vi "upload_session_start.vi"(8 "error in (no error)":errorcluster) -> (0 "error out":errorcluster, 3 "session_id":string)   [LabVIEW 2015, in "lv-dropbox.lvlib" / "v2.lvlib"]
uses:
  v2.lvlib
  private/_controls/content_type.ctl
  <vilib>/httpClient/POSTBuffer.vi
  <vilib>/httpClient/LabVIEWHTTPClient.lvlib
  lv-dropbox.lvlib
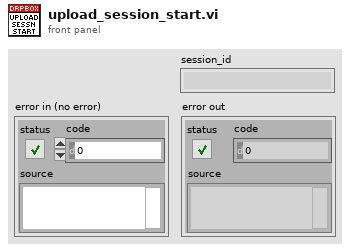
[diagram p1: front panel]
types:
  T1 = typedef "lv-dropbox.lvlib/content_type.ctl" = enum16{"<content_type>", "application/json", "application/octet-stream", "application/x-www-form-urlencoded"}
  T2 = typedef "LabVIEWHTTPClient.lvlib/ClientHandle.ctl" = refnum<k1>
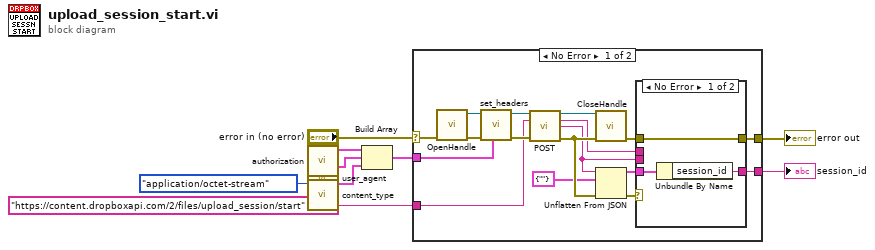
[diagram p0: block diagram]
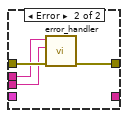
[diagram p2: hidden frame]
diagram:
  n1 = call "authorization.vi"() -> ("header"=w4:cluster{"header":string, "value":string})  [unwired: 11 in]
  n2 = call "user_agent.vi"() -> ("header"=w8:cluster{"header":string, "value":string})  [unwired: 11 in]
  n3 = call "content_type.vi"("content_type"=content_type."application/octet-stream") -> ("header"=w9:cluster{"header":string, "value":string})  [unwired: 10 in]
  n4 = Build Array(w4, w8, w9) -> (w3:cluster{"header":string, "value":string}[])
  n5 = case shown="No Error" "error in (no error)" {
    selector: "error in (no error)" -> [w20 w34]
    tunnel: w3 -> [w18 _]
    tunnel: "https://content.dropboxapi.com/2/files/upload_session/start" ("url") -> [w15 _]
    tunnel: [w10 w34] -> w1
    tunnel: [w16 _] -> w2
    frame No Error {
      n6 = call <vilib>:"OpenHandle.vi"("error in (no error)"=w20) -> ("client handle out"=w23:T2, "error out"=w17:errorcluster)  [unwired: 13 in]
      n7 = call "set_headers.vi"("header_value []"=w18, "error in (no error)"=w17, "client_handle in"=w23) -> ("error out"=w21:errorcluster, "client_handle out"=w22:T2)  [unwired: 7 in]
      n8 = call-poly <vilib>:"POST.vi"("client handle"=w22, "url"=w15, "error in (no error)"=w21) -> ("client handle out"=w24:T2, "headers"=w13:string, "body"=w12:string, "error out"=w26:errorcluster)  [unwired: 9 in]
      n9 = call <vilib>:"CloseHandle.vi"("client handle"=w24, "error in (no error)"=w26) -> ("error out"=w11:errorcluster)  [unwired: 13 in]
      n10 = Unflatten From JSON(JSON string=w12, type and defaults=cluster{"session_id":string} {"session_id"=""} ("value"), error in (no error)=w26) -> (value=w25:cluster{"session_id":string}, error out=w14:errorcluster)  [unwired: 4 in]
      n11 = case shown="No Error" w14 {
        tunnel: w25 -> [w29 _]
        tunnel: [w28 _] -> w16
        tunnel: w13 -> [_ w32]
        tunnel: w12 -> [_ w31]
        tunnel: w11 -> [w27 w33]
        tunnel: [w27 w30] -> w10
        frame No Error {
          n12 = Unbundle By Name(w29) -> ("session_id"=w28:string)
        }
        frame Error {
          n13 = call "error_handler.vi"("error in (no error)"=w33, "body"=w31, "headers"=w32) -> ("error out"=w30:errorcluster)  [unwired: 8 in]
        }
      }
    }
    frame Error {
    }
  }
  "error out" <- w1
  "session_id" <- w2
